vi "氨氮总氮总磷质控流程.vi"(7 "队列输入NH3":refnum<queue>, 8 "总氮":bool, 9 "总磷":bool, 10 "氨氮":bool, 11 "队列输入TP":refnum<queue>) -> (3 "布尔":bool)   [LabVIEW 2016, in "质控单元.lvlib"]
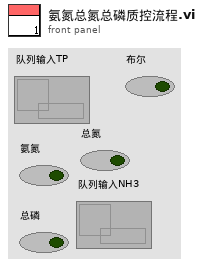
[diagram p1: front panel]
types:
  T1 = enum16{"待机", "启动氨氮水样", "氨氮测量中", "启动氨氮加标", "启动氨氮加标回收", "氨氮加标回收测量中", "启动总氮水样", "总氮测量中", "启动总氮加标", "启动总氮加标回收", "总氮加标回收测量中", "启动总磷水样", "总磷水样测量中", "启动总磷加标", "启动总磷加标回收", "总磷加标回收测量中", "结束"}
  T2 = cluster{"站号":u16, "量程切换":enum32{"H", "L", "AUTO"}, "控制命令":enum16{"启动测量", "标样核查", "零点核查", "跨度核查", "空白测试", "平行样测试", "加标回收", "空白校准", "标样校准", "初始化（清洗）", "停止测试", "仪器重启", "校时", "模式设置", "测量间隔设置"}, "模式设置":enum16{"待机", "连续模式", "周期模式", "定点模式", "受控模式", "手动模式"}, "测量间隔":u16}
  T3 = cluster{"时间标识":timestamp, "设备":string, "日志信息":string}
  T4 = cluster{"系统时间":timestamp, "工作状态":enum16{"空闲", "水样测试", "标样核查", "零点核查", "跨度核查", "空白测试", "平行样测试", "加标回收", "空白校准", "标样校准", "初始化（清洗）"}, "测量模式":enum16{"待机", "连续模式", "周期模式", "定点模式", "受控模式", "手动模式"}, "告警代码":enum16{"无告警", "缺试剂告警", "缺水样告警", "缺蒸馏水告警", "缺标液告警", "仪表漏液告警", "标定异常告警", "超量程告警", "加热异常", "低试剂预警", "超上限告警", "超下限告警", "仪表内部其他异常", "滴定异常告警", "电极异常告警", "量程切换告警", "参数设置告警", "PH电极电位异常", "电导率电极异常", "浊度光度异常", "溶解氧电极异常", "溶解氧光强异常", "温度异常告警", "PH异常告警", "溶解氧异常告警", "电导率异常告警", "浊度异常告警", "叶绿素异常告警", "藻密度异常告警", "蓝绿藻异常告警", "ORP异常告警", "氨氮异常告警", "清洁刷异常告警", "SD卡异常告警", "蓝牙异常告警", "Wifi异常告警", "流程异常告警"}, "故障代码":enum16{"无故障", "电机故障", "温度故障", "通讯故障", "滴定故障"}, "日志代码":u16, "软件版本":u16, "F0":sgl, "F1":sgl, "F2":sgl, "F3":sgl, "T":sgl, "H":sgl, "id":u16, "flowid":u16, "量程":u16}
  T5 = enum16{"空闲", "水样测试", "标样核查", "零点核查", "跨度核查", "空白测试", "平行样测试", "加标回收", "空白校准", "标样校准", "初始化（清洗）"}
  T6 = cluster{"因子编码":u32, "单位":u16, "标样参考值":sgl, "水样数据时间":timestamp, "水样实测值":sgl, "水样数据标识":string, "标样数据时间":timestamp, "标样实测值":sgl, "标样数据标识":string, "空白数据时间":timestamp, "空白实测值":sgl, "空白数据标识":string, "零点核查数据时间":timestamp, "零点核查实测值":sgl, "零点核查数据标识":string, "跨度核查数据时间":timestamp, "跨度核查实测值":sgl, "跨度核查数据标识":string, "加标回收数据时间":timestamp, "加标回收实测值":sgl, "加标回收数据标识":string, "平行样数据时间":timestamp, "平行样实测值":sgl, "平行样数据标识":string}
  T7 = cluster{"量程":dbl, "检出限":dbl, "加标前水样浓度":dbl, "加标后水样浓度":dbl, "加标水杯定容体积":dbl, "加标母液浓度":dbl, "加标体积":dbl, "加标回收率":dbl}
  T8 = cluster{"因子编码":u32, "单位":u16, "标样参考值":sgl, "水样数据时间":timestamp, "水样实测值":sgl, "水样数据标识":string, "标样数据时间":timestamp, "标样实测值":sgl, "标样数据标识":string, "空白数据时间":timestamp, "空白实测值":sgl, "空白数据标识":string, "零点核查数据时间":timestamp, "零点核查实测值":sgl, "零点核查数据标识":string, "跨度核查数据时间":timestamp, "跨度核查实测值":sgl, "跨度核查数据标识":string, "加标回收数据时间":timestamp, "加标回收实测值":sgl, "加标回收数据标识":string, "平行样数据时间":timestamp, "平行样实测值":sgl, "平行样数据标识":string, "F0":sgl, "F1":sgl, "F2":sgl, "F3":sgl, "F4":sgl, "F5":sgl, "F6":sgl, "F7":sgl, "温度":sgl, "湿度":sgl, "X值":sgl}
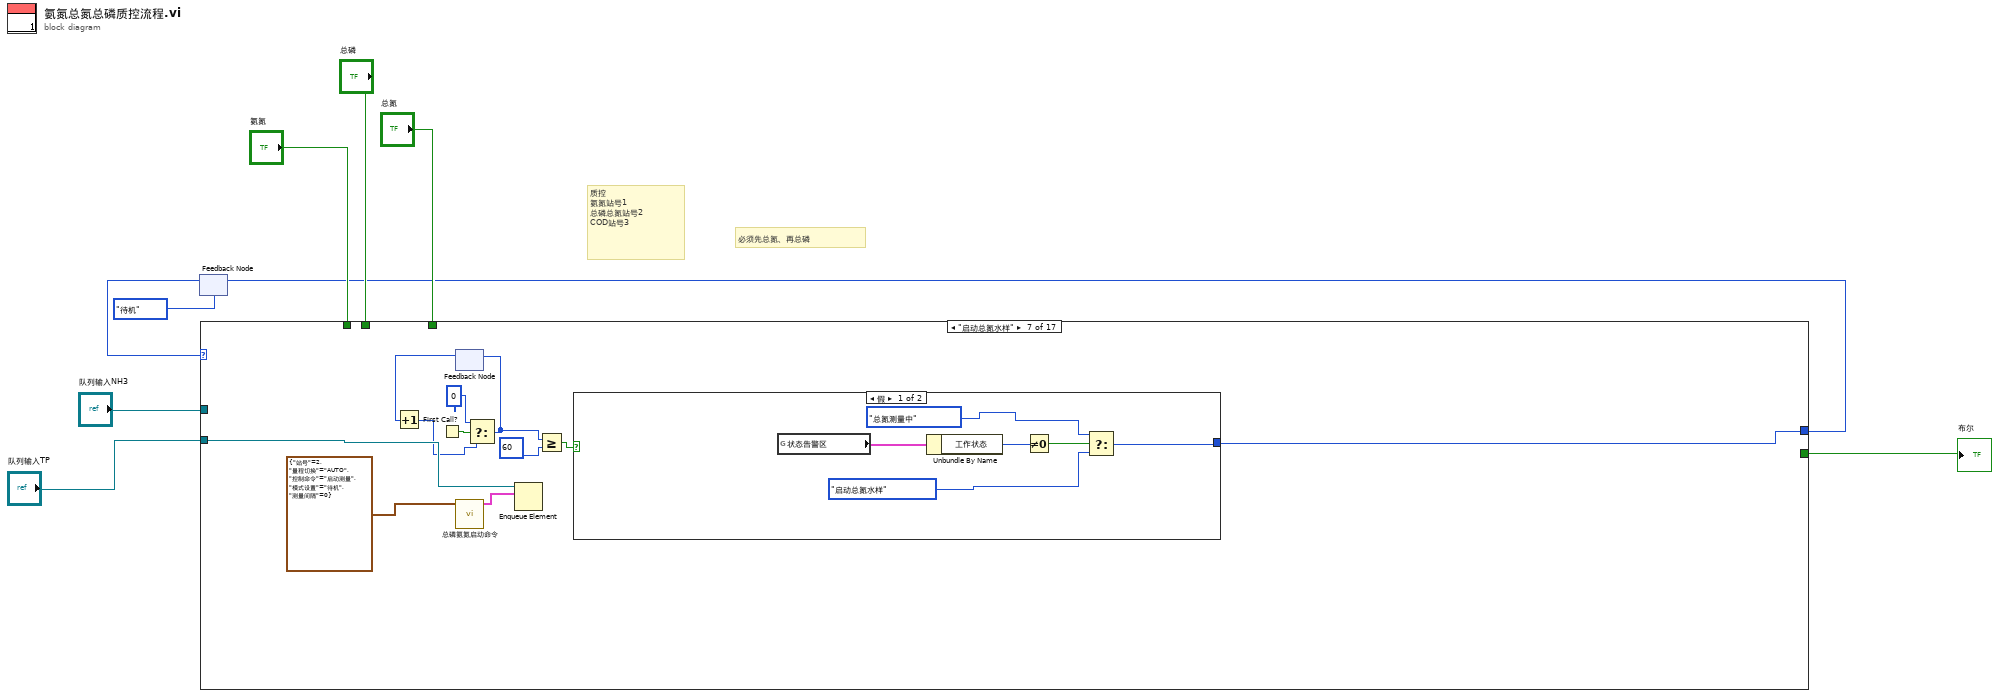
[diagram p0: block diagram]
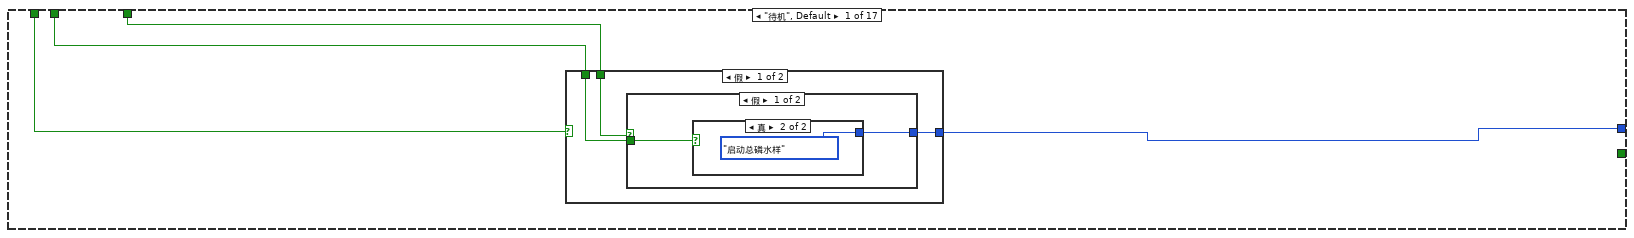
[diagram p2: hidden frame]
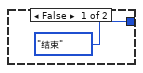
[diagram p3: hidden frame]
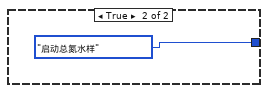
[diagram p4: hidden frame]
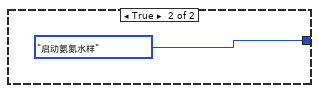
[diagram p5: hidden frame]
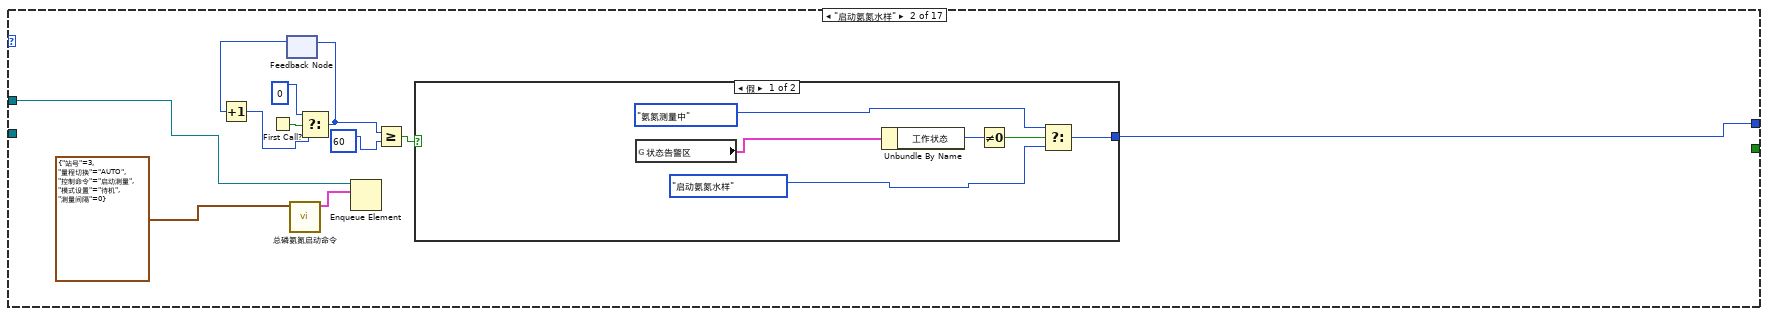
[diagram p6: hidden frame]
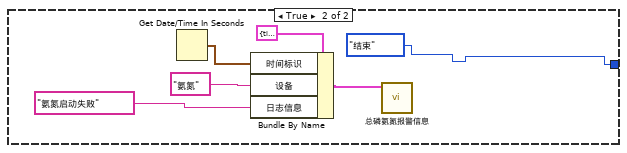
[diagram p7: hidden frame]
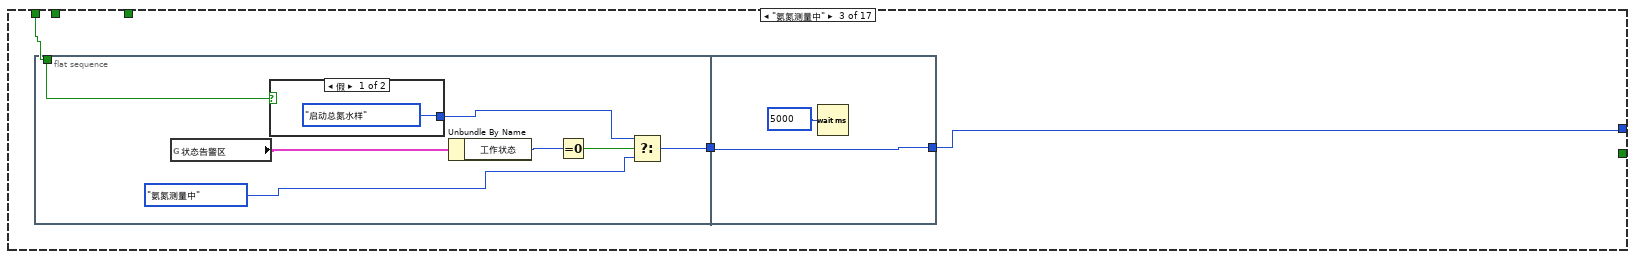
[diagram p8: hidden frame]
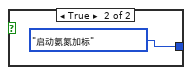
[diagram p9: hidden frame]
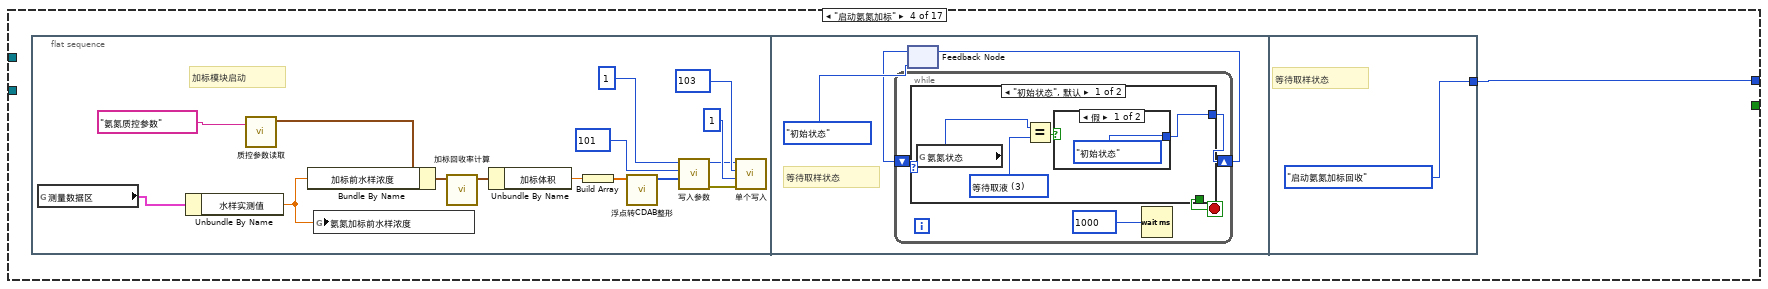
[diagram p10: hidden frame]
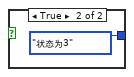
[diagram p11: hidden frame]
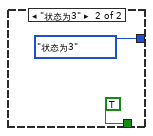
[diagram p12: hidden frame]
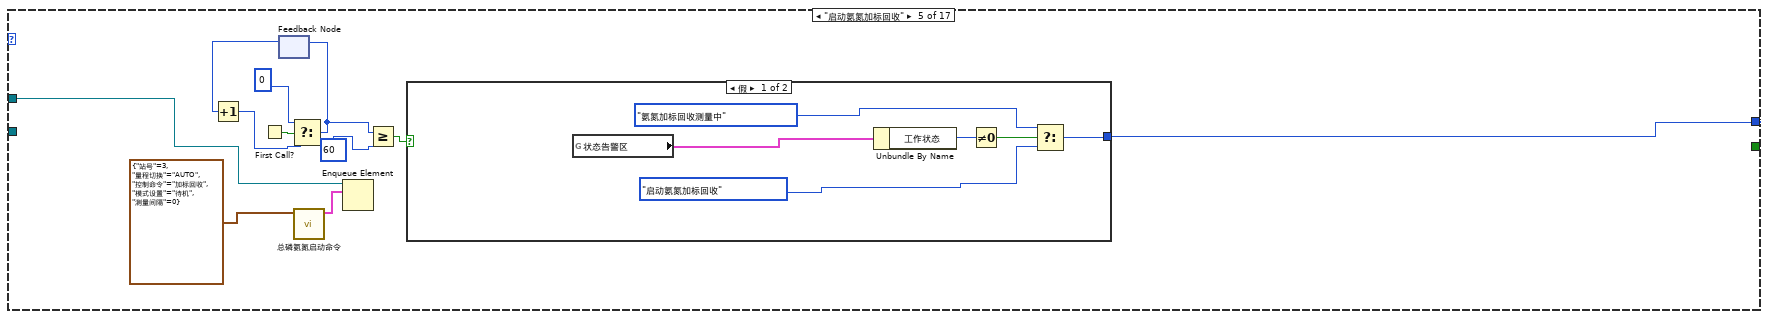
[diagram p13: hidden frame]
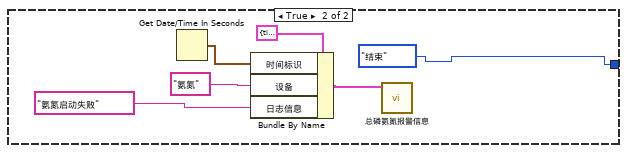
[diagram p14: hidden frame]
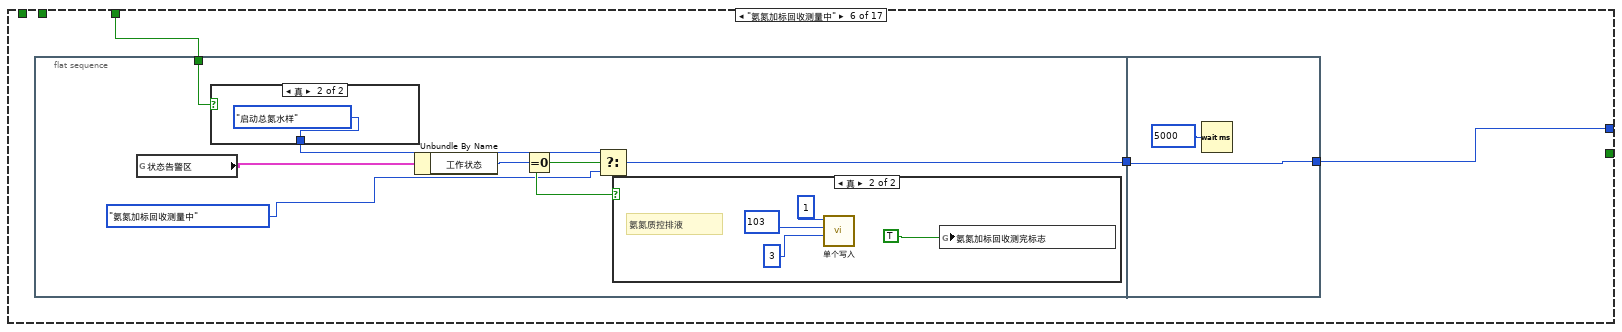
[diagram p15: hidden frame]
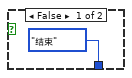
[diagram p16: hidden frame]
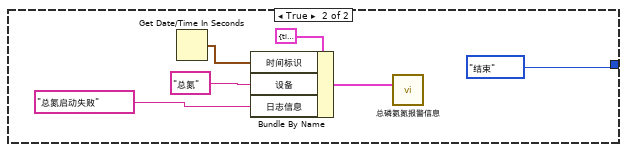
[diagram p18: hidden frame]
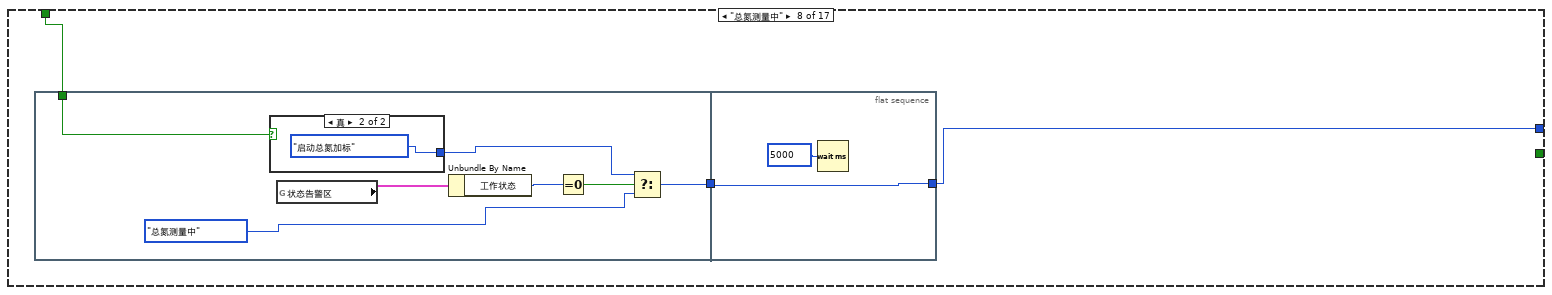
[diagram p19: hidden frame]
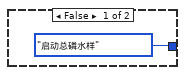
[diagram p20: hidden frame]
diagram:
  # "质控\n氨氮站号1   \n总磷总氮站号2\nCOD站号3"
  # "必须先总氮、再总磷"
  n1 = feedback #1(T1."待机") -> (w4:T1)
  n2 = case shown="\"启动总氮水样\"" w4 {
    tunnel: [w13 w33 w48 w60 w94 w114 w141 w155 w169 w200 w223 w250 w266 w278 w310 w332 T1."结束"] -> w2
    tunnel: "队列输入TP" -> [_ _ _ _ _ _ w142 _ _ w203 _ w251 _ _ w311 _ _]
    tunnel: [_ _ _ _ _ _ _ _ _ _ _ _ _ _ _ _ TRUE] -> w7
    tunnel: "总磷" -> [w11 _ _ _ _ _ _ _ _ _ w224 _ w264 _ _ _ _]
    tunnel: "氨氮" -> [w12 _ w46 _ _ _ _ _ _ _ _ _ _ _ _ _ _]
    tunnel: "总氮" -> [w10 _ _ _ _ w115 _ w156 _ _ _ _ _ _ _ _ _]
    tunnel: "队列输入NH3" -> [_ w23 _ _ w91 _ _ _ _ _ _ _ _ _ _ _ _]
    frame "待机", Default {
      n3 = case shown="假" w12 {
        tunnel: [w15 T1."启动氨氮水样"] -> w13
        tunnel: w11 -> [w16 _]
        tunnel: w10 -> [w14 _]
        frame False {
          n4 = case shown="假" w14 {
            tunnel: w16 -> [w17 _]
            tunnel: [w18 T1."启动总氮水样"] -> w15
            frame False {
              n5 = case shown="真" w17 {
                tunnel: [T1."结束" T1."启动总磷水样"] -> w18
                frame False {
                }
                frame True {
                }
              }
            }
            frame True {
            }
          }
        }
        frame True {
        }
      }
    }
    frame "启动氨氮水样" {
      n6 = First Call?() -> (First Call?: T/F=w31:bool)
      n7 = feedback #2() -> (w30:i32)  [unwired: 1 in]
      n8 = Increment(x=w30) -> (x+1=w29:i32)
      n9 = call "总磷氨氮启动命令.vi"("参数"=T2 {"站号"=3, "量程切换"=enum."AUTO", "控制命令"=enum."启动测量", "模式设置"=enum."待机", "测量间隔"=0}) -> ("启动命令"=w25:cluster{"命令":string, "data":variant})  [unwired: 10 in]
      n10 = Select(t=0, s=w31, f=w29) -> (s? t:f=w28:i32)
      n11 = feedback-in #2(w28) -> ()
      n12 = Enqueue Element(queue=w23, element=w25) -> ()  [unwired: 2 in, 3 out]
      n13 = Greater Or Equal?(x=w28, y=60) -> (x >= y?=w26:bool)
      n14 = case shown="假" w26 {
        tunnel: [w37 T1."结束"] -> w33
        frame False {
          n15 = global read "VAR总磷氨氮全局变量.vi" "状态告警区"() -> (w34:T4)
          n16 = Unbundle By Name(w34) -> ("工作状态"=w39:T5)
          n17 = Not Equal To 0?(x=w39) -> (x != 0?=w38:bool)
          n18 = Select(t=T1."氨氮测量中", s=w38, f=T1."启动氨氮水样") -> (s? t:f=w37:T1)
        }
        frame True {
          n19 = Get Date/Time In Seconds() -> (seconds since 1Jan1904=w45:timestamp)
          n20 = Bundle By Name(cluster=T3 {"时间标识"=timestamp(0 s since 1904-01-01), "设备"="", "日志信息"=""} ("data in"), "时间标识"=w45, "设备"="氨氮", "日志信息"="氨氮启动失败") -> (w41:T3)
          n21 = call "总磷氨氮报警信息.vi"("data in"=w41) -> ()  [unwired: 11 in]
        }
      }
    }
    frame "氨氮测量中" {
      n22 = flat-sequence {
        tunnel: [w54] -> w47
        tunnel: w46 -> [w51]
        tunnel: [w59] -> w48
        tunnel: w47 -> [w59]
        frame #0 {
          n23 = global read "VAR总磷氨氮全局变量.vi" "状态告警区"() -> (w49:T4)
          n24 = case shown="假" w51 {
            tunnel: [T1."启动总氮水样" T1."启动氨氮加标"] -> w52
            frame False {
            }
            frame True {
            }
          }
          n25 = Unbundle By Name(w49) -> ("工作状态"=w55:T5)
          n26 = Equal To 0?(x=w55) -> (x = 0?=w53:bool)
          n27 = Select(t=w52, s=w53, f=T1."氨氮测量中") -> (s? t:f=w54:T1)
        }
        frame #1 {
          n28 = Wait (ms)(milliseconds to wait=u32 5000 ("等待时间（毫秒）")) -> ()  [unwired: 1 out]
        }
      }
    }
    frame "启动氨氮加标" {
      n29 = flat-sequence {
        tunnel: [T1."启动氨氮加标回收"] -> w60
        frame #0 {
          w64 = u16 1 ("value")
          # "加标模块启动"
          n30 = global read "VAR总磷氨氮全局变量.vi" "测量数据区"() -> (w61:T6)
          n31 = Unbundle By Name(w61) -> ("水样实测值"=w62:sgl)
          n32 = call "质控参数读取.vi"("section"="氨氮质控参数") -> ("参数"=w72:T7)  [unwired: 9 in, 1 out]
          n33 = Bundle By Name(cluster=w72, "加标前水样浓度"=w62) -> (w73:T7)
          n34 = global write "水样浓度全局.vi" "氨氮加标前水样浓度"(w62) -> ()
          n35 = call "加标回收率计算.vi"("参数"=w73) -> ("参数 out"=w71:T7)  [unwired: 10 in]
          n36 = Unbundle By Name(w71) -> ("加标体积"=w63:dbl)
          n37 = Build Array(w63) -> (w70:dbl[])
          n38 = call "浮点转CDAB整形.vi"("浮点数"=w70) -> ("CDAB整形输出"=w65:u16[])  [unwired: 10 in]
          n39 = call "写入参数.vi"("values"=w65, "starting address"=u16 101, "Slave ID"=w64) -> ("error out"=w69:errorcluster)  [unwired: 8 in]
          n40 = call "单个写入.vi"("Error in"=w69, "value"=u16 1, "address"=u16 103, "Slave ID"=w64) -> ()  [unwired: 7 in, 1 out]
        }
        frame #1 {
          # "等待取样状态"
          n41 = feedback #3(enum16{"初始状态", "状态为3"}."初始状态") -> (w76:enum16{"初始状态", "状态为3"})
          n42 = while {
            shift-right: [w80] -> w75
            shift-left: w76 -> [w81]
            stop <- w79 stop-if-true
            n43 = case shown="\"初始状态\", 默认" w81 {
              tunnel: [w83 enum16{"初始状态", "状态为3"}."状态为3"] -> w80
              tunnel: [_ TRUE] -> w79
              frame "初始状态", Default {
                w82 = u16 3 items=["待机", "润洗", "进样", "等待取液", "排液"] ("氨氮状态")
                n44 = global read "氨氮加标回收状态全局变量.vi" "氨氮状态"() -> (w85:u16)
                n45 = Equal?(x=w85, y=w82) -> (x = y?=w84:bool)
                n46 = case shown="假" w84 {
                  tunnel: [enum16{"初始状态", "状态为3"}."初始状态" enum16{"初始状态", "状态为3"}."状态为3"] -> w83
                  frame False {
                  }
                  frame True {
                  }
                }
              }
              frame "状态为3" {
              }
            }
            n47 = Wait (ms)(milliseconds to wait=u32 1000 ("等待时间（毫秒）")) -> ()  [unwired: 1 out]
          }
          n48 = feedback-in #3(w75) -> ()
        }
        frame #2 {
          # "等待取样状态"
        }
      }
    }
    frame "启动氨氮加标回收" {
      n49 = First Call?() -> (First Call?: T/F=w100:bool)
      n50 = feedback #4() -> (w99:i32)  [unwired: 1 in]
      n51 = Increment(x=w99) -> (x+1=w98:i32)
      n52 = Select(t=0, s=w100, f=w98) -> (s? t:f=w97:i32)
      n53 = feedback-in #4(w97) -> ()
      n54 = call "总磷氨氮启动命令.vi"("参数"=T2 {"站号"=3, "量程切换"=enum."AUTO", "控制命令"=enum."加标回收", "模式设置"=enum."待机", "测量间隔"=0}) -> ("启动命令"=w93:cluster{"命令":string, "data":variant})  [unwired: 10 in]
      n55 = Enqueue Element(queue=w91, element=w93) -> ()  [unwired: 2 in, 3 out]
      n56 = Greater Or Equal?(x=w97, y=60) -> (x >= y?=w95:bool)
      n57 = case shown="假" w95 {
        tunnel: [w105 T1."结束"] -> w94
        frame False {
          n58 = global read "VAR总磷氨氮全局变量.vi" "状态告警区"() -> (w102:T4)
          n59 = Unbundle By Name(w102) -> ("工作状态"=w107:T5)
          n60 = Not Equal To 0?(x=w107) -> (x != 0?=w106:bool)
          n61 = Select(t=T1."氨氮加标回收测量中", s=w106, f=T1."启动氨氮加标回收") -> (s? t:f=w105:T1)
        }
        frame True {
          n62 = Get Date/Time In Seconds() -> (seconds since 1Jan1904=w113:timestamp)
          n63 = Bundle By Name(cluster=T3 {"时间标识"=timestamp(0 s since 1904-01-01), "设备"="", "日志信息"=""} ("data in"), "时间标识"=w113, "设备"="氨氮", "日志信息"="氨氮启动失败") -> (w109:T3)
          n64 = call "总磷氨氮报警信息.vi"("data in"=w109) -> ()  [unwired: 11 in]
        }
      }
    }
    frame "氨氮加标回收测量中" {
      n65 = flat-sequence {
        tunnel: [w122] -> w116
        tunnel: w115 -> [w119]
        tunnel: [w131] -> w114
        tunnel: w116 -> [w131]
        frame #0 {
          n66 = global read "VAR总磷氨氮全局变量.vi" "状态告警区"() -> (w117:T4)
          n67 = case shown="真" w119 {
            tunnel: [T1."结束" T1."启动总氮水样"] -> w121
            frame False {
            }
            frame True {
            }
          }
          n68 = Unbundle By Name(w117) -> ("工作状态"=w123:T5)
          n69 = Equal To 0?(x=w123) -> (x = 0?=w120:bool)
          n70 = Select(t=w121, s=w120, f=T1."氨氮加标回收测量中") -> (s? t:f=w122:T1)
          n71 = case shown="真" w120 {
            frame False {
            }
            frame True {
              # "氨氮质控排液"
              n72 = call "单个写入.vi"("value"=u16 3, "address"=u16 103, "Slave ID"=u8 1) -> ()  [unwired: 8 in, 1 out]
              n73 = global write "质控测完标志全局 1.vi" "氨氮加标回收测完标志"(TRUE) -> ()
            }
          }
        }
        frame #1 {
          n74 = Wait (ms)(milliseconds to wait=u32 5000 ("等待时间（毫秒）")) -> ()  [unwired: 1 out]
        }
      }
    }
    frame "启动总氮水样" {
      n75 = First Call?() -> (First Call?: T/F=w139:bool)
      n76 = feedback #5() -> (w138:i32)  [unwired: 1 in]
      n77 = Increment(x=w138) -> (x+1=w137:i32)
      n78 = call "总磷氨氮启动命令.vi"("参数"=T2 {"站号"=2, "量程切换"=enum."AUTO", "控制命令"=enum."启动测量", "模式设置"=enum."待机", "测量间隔"=0}) -> ("启动命令"=w133:cluster{"命令":string, "data":variant})  [unwired: 10 in]
      n79 = Select(t=0, s=w139, f=w137) -> (s? t:f=w136:i32)
      n80 = feedback-in #5(w136) -> ()
      n81 = Enqueue Element(queue=w142, element=w133) -> ()  [unwired: 2 in, 3 out]
      n82 = Greater Or Equal?(x=w136, y=60) -> (x >= y?=w134:bool)
      n83 = case shown="假" w134 {
        tunnel: [w145 T1."结束"] -> w141
        frame False {
          n84 = global read "VAR总磷氨氮全局变量.vi" "状态告警区"() -> (w146:T4)
          n85 = Unbundle By Name(w146) -> ("工作状态"=w147:T5)
          n86 = Not Equal To 0?(x=w147) -> (x != 0?=w148:bool)
          n87 = Select(t=T1."总氮测量中", s=w148, f=T1."启动总氮水样") -> (s? t:f=w145:T1)
        }
        frame True {
          n88 = Get Date/Time In Seconds() -> (seconds since 1Jan1904=w154:timestamp)
          n89 = Bundle By Name(cluster=T3 {"时间标识"=timestamp(0 s since 1904-01-01), "设备"="", "日志信息"=""} ("data in"), "时间标识"=w154, "设备"="总氮", "日志信息"="总氮启动失败") -> (w150:T3)
          n90 = call "总磷氨氮报警信息.vi"("data in"=w150) -> ()  [unwired: 11 in]
        }
      }
    }
    frame "总氮测量中" {
      n91 = flat-sequence {
        tunnel: [w162] -> w157
        tunnel: w156 -> [w159]
        tunnel: [w168] -> w155
        tunnel: w157 -> [w168]
        frame #0 {
          n92 = case shown="真" w159 {
            tunnel: [T1."启动总磷水样" T1."启动总氮加标"] -> w160
            frame False {
            }
            frame True {
            }
          }
          n93 = global read "VAR总磷氨氮全局变量.vi" "状态告警区"() -> (w163:T4)
          n94 = Unbundle By Name(w163) -> ("工作状态"=w164:T5)
          n95 = Equal To 0?(x=w164) -> (x = 0?=w161:bool)
          n96 = Select(t=w160, s=w161, f=T1."总氮测量中") -> (s? t:f=w162:T1)
        }
        frame #1 {
          n97 = Wait (ms)(milliseconds to wait=u32 5000 ("等待时间（毫秒）")) -> ()  [unwired: 1 out]
        }
      }
    }
    frame "启动总氮加标" {
      n98 = flat-sequence {
        tunnel: [T1."启动总氮加标回收"] -> w169
        frame #0 {
          w174 = u16 2 ("value")
          # "加标模块启动"
          n99 = global read "VAR总磷氨氮全局变量.vi" "测量数据区"() -> (w172:T8)
          n100 = Unbundle By Name(w172) -> ("水样实测值"=w170:sgl)
          n101 = call "质控参数读取.vi"("section"="总氮质控参数") -> ("参数"=w171:T7)  [unwired: 9 in, 1 out]
          n102 = Bundle By Name(cluster=w171, "加标前水样浓度"=w170) -> (w182:T7)
          n103 = global write "水样浓度全局.vi" "总氮加标前水样浓度"(w170) -> ()
          n104 = call "加标回收率计算.vi"("参数"=w182) -> ("参数 out"=w181:T7)  [unwired: 10 in]
          n105 = Unbundle By Name(w181) -> ("加标体积"=w173:dbl)
          n106 = Build Array(w173) -> (w180:dbl[])
          n107 = call "浮点转CDAB整形.vi"("浮点数"=w180) -> ("CDAB整形输出"=w175:u16[])  [unwired: 10 in]
          n108 = call "写入参数.vi"("values"=w175, "starting address"=u16 101, "Slave ID"=w174) -> ("error out"=w179:errorcluster)  [unwired: 8 in]
          n109 = call "单个写入.vi"("Error in"=w179, "value"=u16 2, "address"=u16 103, "Slave ID"=w174) -> ()  [unwired: 7 in, 1 out]
        }
        frame #1 {
          # "等待取样状态"
          n110 = feedback #6(enum16{"初始状态", "状态为3"}."初始状态") -> (w185:enum16{"初始状态", "状态为3"})
          n111 = while {
            shift-right: [w189] -> w184
            shift-left: w185 -> [w190]
            stop <- w188 stop-if-true
            n112 = case shown="\"状态为3\"" w190 {
              tunnel: [w191 enum16{"初始状态", "状态为3"}."状态为3"] -> w189
              tunnel: [_ TRUE] -> w188
              frame "初始状态", Default {
                n113 = global read "氨氮加标回收状态全局变量.vi" "总磷状态"() -> (w193:u16)
                n114 = Equal?(x=w193, y=u16 3) -> (x = y?=w192:bool)
                n115 = case shown="真" w192 {
                  tunnel: [enum16{"初始状态", "状态为3"}."初始状态" enum16{"初始状态", "状态为3"}."状态为3"] -> w191
                  frame False {
                  }
                  frame True {
                  }
                }
              }
              frame "状态为3" {
              }
            }
            n116 = Wait (ms)(milliseconds to wait=u32 1000 ("等待时间（毫秒）")) -> ()  [unwired: 1 out]
          }
          n117 = feedback-in #6(w184) -> ()
        }
        frame #2 {
          # "等待取样状态"
        }
      }
    }
    frame "启动总氮加标回收" {
      n118 = First Call?() -> (First Call?: T/F=w209:bool)
      n119 = feedback #7() -> (w208:i32)  [unwired: 1 in]
      n120 = Increment(x=w208) -> (x+1=w207:i32)
      n121 = call "总磷氨氮启动命令.vi"("参数"=T2 {"站号"=2, "量程切换"=enum."AUTO", "控制命令"=enum."加标回收", "模式设置"=enum."待机", "测量间隔"=0}) -> ("启动命令"=w201:cluster{"命令":string, "data":variant})  [unwired: 10 in]
      n122 = Select(t=0, s=w209, f=w207) -> (s? t:f=w206:i32)
      n123 = feedback-in #7(w206) -> ()
      n124 = Enqueue Element(queue=w203, element=w201) -> ()  [unwired: 2 in, 3 out]
      n125 = Greater Or Equal?(x=w206, y=60) -> (x >= y?=w204:bool)
      n126 = case shown="假" w204 {
        tunnel: [w213 T1."结束"] -> w200
        frame False {
          n127 = global read "VAR总磷氨氮全局变量.vi" "状态告警区"() -> (w216:T4)
          n128 = Unbundle By Name(w216) -> ("工作状态"=w215:T5)
          n129 = Not Equal To 0?(x=w215) -> (x != 0?=w214:bool)
          n130 = Select(t=T1."总氮加标回收测量中", s=w214, f=T1."启动总氮加标回收") -> (s? t:f=w213:T1)
        }
        frame True {
          n131 = Get Date/Time In Seconds() -> (seconds since 1Jan1904=w222:timestamp)
          n132 = Bundle By Name(cluster=T3 {"时间标识"=timestamp(0 s since 1904-01-01), "设备"="", "日志信息"=""} ("data in"), "时间标识"=w222, "设备"="氨氮", "日志信息"="氨氮启动失败") -> (w218:T3)
          n133 = call "总磷氨氮报警信息.vi"("data in"=w218) -> ()  [unwired: 11 in]
        }
      }
    }
    frame "总氮加标回收测量中" {
      n134 = flat-sequence {
        tunnel: [w230] -> w225
        tunnel: w224 -> [w227]
        tunnel: [w240] -> w223
        tunnel: w225 -> [w240]
        frame #0 {
          n135 = case shown="真" w227 {
            tunnel: [T1."结束" T1."启动总磷水样"] -> w229
            frame False {
            }
            frame True {
            }
          }
          n136 = global read "VAR总磷氨氮全局变量.vi" "状态告警区"() -> (w231:T4)
          n137 = Unbundle By Name(w231) -> ("工作状态"=w232:T5)
          n138 = Equal To 0?(x=w232) -> (x = 0?=w228:bool)
          n139 = Select(t=w229, s=w228, f=T1."总氮加标回收测量中") -> (s? t:f=w230:T1)
          n140 = case shown="真" w228 {
            frame False {
            }
            frame True {
              # "总氮质控排液"
              n141 = call "单个写入.vi"("value"=u16 3, "address"=u16 103, "Slave ID"=u8 2) -> ()  [unwired: 8 in, 1 out]
              n142 = global write "质控测完标志全局 1.vi" "总氮加标回收测完标志"(TRUE) -> ()
            }
          }
        }
        frame #1 {
          n143 = Wait (ms)(milliseconds to wait=u32 5000 ("等待时间（毫秒）")) -> ()  [unwired: 1 out]
        }
      }
    }
    frame "启动总磷水样" {
      n144 = First Call?() -> (First Call?: T/F=w248:bool)
      n145 = feedback #8() -> (w247:i32)  [unwired: 1 in]
      n146 = Increment(x=w247) -> (x+1=w246:i32)
      n147 = call "总磷氨氮启动命令.vi"("参数"=T2 {"站号"=1, "量程切换"=enum."AUTO", "控制命令"=enum."启动测量", "模式设置"=enum."待机", "测量间隔"=0}) -> ("启动命令"=w242:cluster{"命令":string, "data":variant})  [unwired: 10 in]
      n148 = Select(t=0, s=w248, f=w246) -> (s? t:f=w245:i32)
      n149 = feedback-in #8(w245) -> ()
      n150 = Enqueue Element(queue=w251, element=w242) -> ()  [unwired: 2 in, 3 out]
      n151 = Greater Or Equal?(x=w245, y=60) -> (x >= y?=w243:bool)
      n152 = case shown="假" w243 {
        tunnel: [w254 T1."结束"] -> w250
        frame False {
          n153 = global read "VAR总磷氨氮全局变量.vi" "状态告警区"() -> (w255:T4)
          n154 = Unbundle By Name(w255) -> ("工作状态"=w256:T5)
          n155 = Not Equal To 0?(x=w256) -> (x != 0?=w257:bool)
          n156 = Select(t=T1."总磷水样测量中", s=w257, f=T1."启动总磷水样") -> (s? t:f=w254:T1)
        }
        frame True {
          n157 = Get Date/Time In Seconds() -> (seconds since 1Jan1904=w263:timestamp)
          n158 = Bundle By Name(cluster=T3 {"时间标识"=timestamp(0 s since 1904-01-01), "设备"="", "日志信息"=""} ("data in"), "时间标识"=w263, "设备"="总磷", "日志信息"="总磷启动失败") -> (w259:T3)
          n159 = call "总磷氨氮报警信息.vi"("data in"=w259) -> ()  [unwired: 11 in]
        }
      }
    }
    frame "总磷水样测量中" {
      n160 = flat-sequence {
        tunnel: [w271] -> w265
        tunnel: w264 -> [w268]
        tunnel: [w277] -> w266
        tunnel: w265 -> [w277]
        frame #0 {
          n161 = case shown="真" w268 {
            tunnel: [T1."结束" T1."启动总磷加标"] -> w269
            frame False {
            }
            frame True {
            }
          }
          n162 = global read "VAR总磷氨氮全局变量.vi" "状态告警区"() -> (w272:T4)
          n163 = Unbundle By Name(w272) -> ("工作状态"=w273:T5)
          n164 = Equal To 0?(x=w273) -> (x = 0?=w270:bool)
          n165 = Select(t=w269, s=w270, f=T1."总磷水样测量中") -> (s? t:f=w271:T1)
        }
        frame #1 {
          n166 = Wait (ms)(milliseconds to wait=u32 5000 ("等待时间（毫秒）")) -> ()  [unwired: 1 out]
        }
      }
    }
    frame "启动总磷加标" {
      n167 = flat-sequence {
        tunnel: [T1."启动总磷加标回收"] -> w278
        frame #0 {
          w283 = u16 2 ("value")
          # "加标模块启动"
          n168 = global read "VAR总磷氨氮全局变量.vi" "测量数据区"() -> (w281:T8)
          n169 = Unbundle By Name(w281) -> ("水样实测值"=w279:sgl)
          n170 = call "质控参数读取.vi"("section"="总磷质控参数") -> ("参数"=w280:T7)  [unwired: 9 in, 1 out]
          n171 = Bundle By Name(cluster=w280, "加标前水样浓度"=w279) -> (w291:T7)
          n172 = global write "水样浓度全局.vi" "总磷加标前水样浓度"(w279) -> ()
          n173 = call "加标回收率计算.vi"("参数"=w291) -> ("参数 out"=w290:T7)  [unwired: 10 in]
          n174 = Unbundle By Name(w290) -> ("加标体积"=w282:dbl)
          n175 = Build Array(w282) -> (w289:dbl[])
          n176 = call "浮点转CDAB整形.vi"("浮点数"=w289) -> ("CDAB整形输出"=w284:u16[])  [unwired: 10 in]
          n177 = call "写入参数.vi"("values"=w284, "starting address"=u16 101, "Slave ID"=w283) -> ("error out"=w288:errorcluster)  [unwired: 8 in]
          n178 = call "单个写入.vi"("Error in"=w288, "value"=u16 2, "address"=u16 103, "Slave ID"=w283) -> ()  [unwired: 7 in, 1 out]
        }
        frame #1 {
          # "等待取样状态"
          n179 = feedback #9(enum16{"初始状态", "状态为3"}."初始状态") -> (w294:enum16{"初始状态", "状态为3"})
          n180 = while {
            shift-right: [w298] -> w293
            shift-left: w294 -> [w299]
            stop <- w297 stop-if-true
            n181 = case shown="\"状态为3\"" w299 {
              tunnel: [w300 enum16{"初始状态", "状态为3"}."状态为3"] -> w298
              tunnel: [_ TRUE] -> w297
              frame "初始状态", Default {
                n182 = global read "氨氮加标回收状态全局变量.vi" "总磷状态"() -> (w302:u16)
                n183 = Equal?(x=w302, y=u16 3) -> (x = y?=w301:bool)
                n184 = case shown="真" w301 {
                  tunnel: [enum16{"初始状态", "状态为3"}."初始状态" enum16{"初始状态", "状态为3"}."状态为3"] -> w300
                  frame False {
                  }
                  frame True {
                  }
                }
              }
              frame "状态为3" {
              }
            }
            n185 = Wait (ms)(milliseconds to wait=u32 1000 ("等待时间（毫秒）")) -> ()  [unwired: 1 out]
          }
          n186 = feedback-in #9(w293) -> ()
        }
        frame #2 {
          # "等待取样状态"
        }
      }
    }
    frame "启动总磷加标回收" {
      n187 = First Call?() -> (First Call?: T/F=w318:bool)
      n188 = feedback #10() -> (w317:i32)  [unwired: 1 in]
      n189 = Increment(x=w317) -> (x+1=w316:i32)
      n190 = call "总磷氨氮启动命令.vi"("参数"=T2 {"站号"=1, "量程切换"=enum."AUTO", "控制命令"=enum."加标回收", "模式设置"=enum."待机", "测量间隔"=0}) -> ("启动命令"=w312:cluster{"命令":string, "data":variant})  [unwired: 10 in]
      n191 = Select(t=0, s=w318, f=w316) -> (s? t:f=w315:i32)
      n192 = feedback-in #10(w315) -> ()
      n193 = Enqueue Element(queue=w311, element=w312) -> ()  [unwired: 2 in, 3 out]
      n194 = Greater Or Equal?(x=w315, y=60) -> (x >= y?=w313:bool)
      n195 = case shown="真" w313 {
        tunnel: [w322 T1."结束"] -> w310
        frame False {
          n196 = global read "VAR总磷氨氮全局变量.vi" "状态告警区"() -> (w323:T4)
          n197 = Unbundle By Name(w323) -> ("工作状态"=w324:T5)
          n198 = Not Equal To 0?(x=w324) -> (x != 0?=w325:bool)
          n199 = Select(t=T1."总磷加标回收测量中", s=w325, f=T1."启动总磷加标回收") -> (s? t:f=w322:T1)
        }
        frame True {
          n200 = Get Date/Time In Seconds() -> (seconds since 1Jan1904=w331:timestamp)
          n201 = Bundle By Name(cluster=T3 {"时间标识"=timestamp(0 s since 1904-01-01), "设备"="", "日志信息"=""} ("data in"), "时间标识"=w331, "设备"="总磷", "日志信息"="总磷启动失败") -> (w327:T3)
          n202 = call "总磷氨氮报警信息.vi"("data in"=w327) -> ()  [unwired: 11 in]
        }
      }
    }
    frame "总磷加标回收测量中" {
      n203 = flat-sequence {
        tunnel: [w337] -> w333
        tunnel: [w345] -> w332
        tunnel: w333 -> [w345]
        frame #0 {
          n204 = global read "VAR总磷氨氮全局变量.vi" "状态告警区"() -> (w338:T4)
          n205 = Unbundle By Name(w338) -> ("工作状态"=w339:T5)
          n206 = Equal To 0?(x=w339) -> (x = 0?=w336:bool)
          n207 = Select(t=T1."结束", s=w336, f=T1."总磷加标回收测量中") -> (s? t:f=w337:T1)
          n208 = case shown="真" w336 {
            frame False {
            }
            frame True {
              # "总磷质控排液"
              n209 = global write "质控测完标志全局 1.vi" "总磷加标回收测完标志"(TRUE) -> ()
              n210 = call "单个写入.vi"("value"=u16 3, "address"=u16 103, "Slave ID"=u8 2) -> ()  [unwired: 8 in, 1 out]
            }
          }
        }
        frame #1 {
          n211 = Wait (ms)(milliseconds to wait=u32 5000 ("等待时间（毫秒）")) -> ()  [unwired: 1 out]
        }
      }
    }
    frame "结束" {
    }
  }
  "布尔" <- w7
  n212 = feedback-in #1(w2) -> ()
